vi "MGCC_FntStaMach_Flagtoevent.vi"(9 "M_OFF":bool, 10 "Pre_state":string) -> (2 "Event":bool[](array[boolean]))   [LabVIEW 2016]
uses:
  <vilib>/imath/engines/lvmath/Plug In/_Char/NIMS_CH_character datatype.ctl
  <vilib>/imath/engines/lvmath/Plug In/_Char/NIMS_CH_String to Character Array.vi
  <vilib>/imath/engines/lvmath2/RunTimeEngine/IndexRead/NIMS V(S).vi
  <instcachedir>/0/NIMS V(S)_0488751826AF41519A22953C041130DC.lvgen/NIMS V(S)_0488751826AF41519A22953C041130DC_003.vi
  <vilib>/imath/engines/lvmath2/RunTimeEngine/ErrorHandling/NIMS_Create Error From Enums.vi
  <vilib>/imathl/engines/lvmath/Functions/Error Handling/Create Error.vi
  <vilib>/imath/engines/lvmath2/RunTimeSupport/NIMS_Compare Aggregates.vi
  <instcachedir>/0/NIMS_Compare Aggregates_FA3EBEB3749E48D38A57888B5ABBF163.lvgen/NIMS_Compare Aggregates_FA3EBEB3749E48D38A57888B5ABBF163_000.vi
  <vilib>/imath/engines/lvmath2/RunTimeEngine/VariableToken/NIMS_VariableToken_CondDefined.vi
  <instcachedir>/0/NIMS_VariableToken_CondDefined_06E9DA95BD4D46A6BA55EC651A891960.lvgen/NIMS_VariableToken_CondDefined_06E9DA95BD4D46A6BA55EC651A891960_003.vi
  <vilib>/imath/engines/lvmath2/RunTimeEngine/NodeEndStatement/NIMS_NodeEndStatement_Output.vi
  <instcachedir>/0/NIMS_NodeEndStatement_Output_53EC0D466D134D7ABD903AC30B43404B.lvgen/NIMS_NodeEndStatement_Output_53EC0D466D134D7ABD903AC30B43404B_012.vi
  <vilib>/imath/engines/lvmath2/RunTimeEngine/ErrorHandling/NIMS_Finalize Error.vi
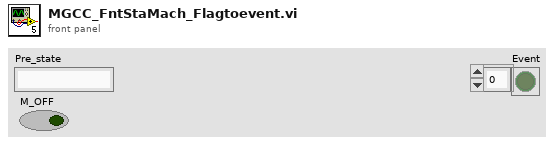
[diagram p1: front panel]
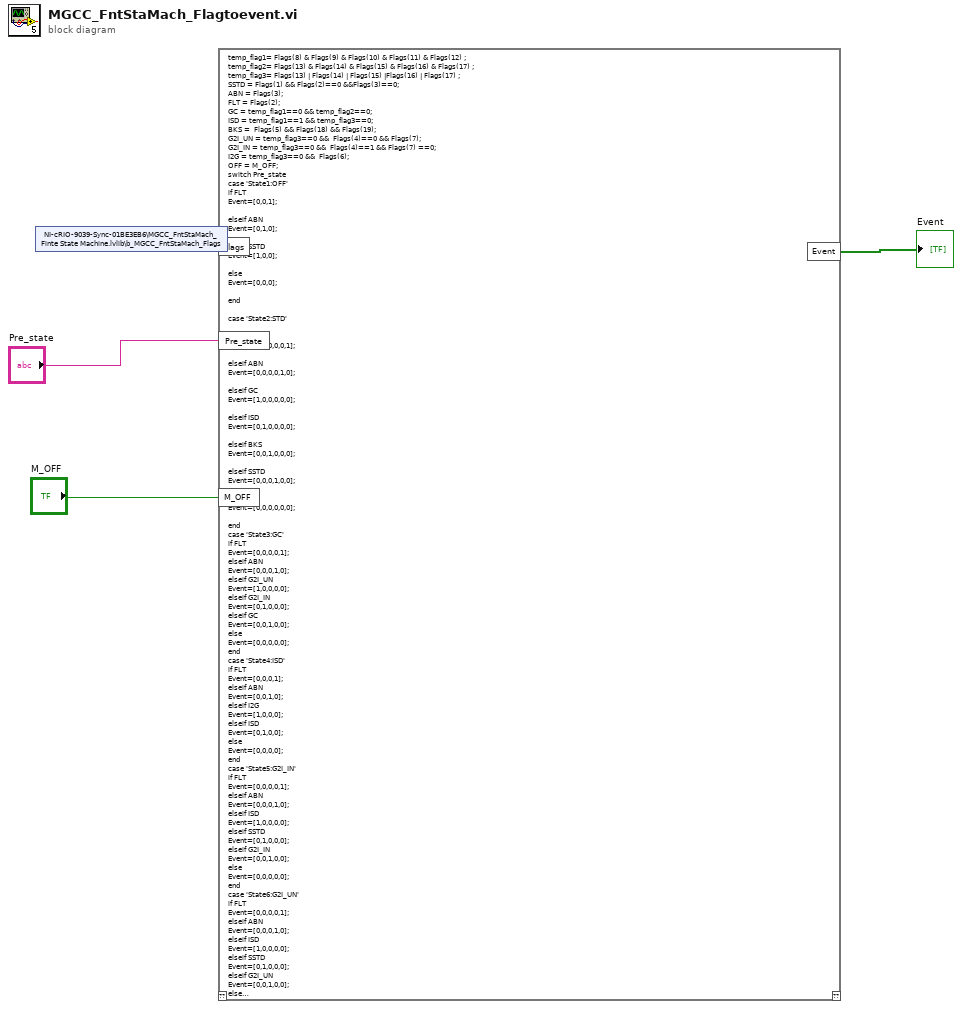
[diagram p0: block diagram]
diagram:
  n1 = shared-variable "NI-cRIO-9039-Sync-01BE3EB6\\MGCC_FntStaMach_Finte State Machine.lvlib\\b_MGCC_FntStaMach_Flags"() -> (w4:bool[])  [unwired: 1 in, 1 out]
  n2 = mathscript code="temp_flag1= Flags(8) & Flags(9) & Flags(10) & Flags(11) & Flags(12) ;\ntemp_flag2= Flags(13) & Flags(14) & Flags(15) & Flags(16) & Flags(17) ;\ntemp_flag3= Flags(13) | Flags(14) | Flags(15) |Flags(16) | Flags(17) ;\nSSTD = Flags(1) && Flags(2)==0 &&Flags(3)==0;\nABN = Flags(3);\nFLT = Flags(2);\nGC = temp_flag1==0 && temp_flag2==0;\nISD = temp_flag1==1 && temp_flag3==0;\nBKS =  Flags(5) && Flags(18) && Flags(19);\nG2I_UN = temp_flag3==0 &&  Flags(4)==0 && Flags(7);\nG2I_IN = temp_flag3==0 &&  Flags(4)==1 && Flags(7) ==0;\nI2G = temp_flag3==0 &&  Flags(6);\nOFF = M_OFF;\nswitch Pre_state\ncase 'State1:OFF'\nif FLT\nEvent=[0,0,1];\n\nelseif ABN\nEvent=[0,1,0];\n\nelseif SSTD\nEvent=[1,0,0];\n\nelse\nEvent=[0,0,0];\n\nend \n\ncase 'State2:STD'\n\nif FLT\nEvent=[0,0,0,0,0,1];\n\nelseif ABN\nEvent=[0,0,0,0,1,0];\n\nelseif GC\nEvent=[1,0,0,0,0,0];\n\nelseif ISD\nEvent=[0,1,0,0,0,0];\n\nelseif BKS\nEvent=[0,0,1,0,0,0];\n\nelseif SSTD\nEvent=[0,0,0,1,0,0];\n\nelse\nEvent=[0,0,0,0,0,0];\n\nend \ncase 'State3:GC'\nif FLT\nEvent=[0,0,0,0,1];\nelseif ABN\nEvent=[0,0,0,1,0];\nelseif G2I_UN\nEvent=[1,0,0,0,0];\nelseif G2I_IN\nEvent=[0,1,0,0,0];\nelseif GC\nEvent=[0,0,1,0,0];\nelse\nEvent=[0,0,0,0,0];\nend\ncase 'State4:ISD'\nif FLT\nEvent=[0,0,0,1];\nelseif ABN\nEvent=[0,0,1,0];\nelseif I2G\nEvent=[1,0,0,0];\nelseif ISD\nEvent=[0,1,0,0];\nelse\nEvent=[0,0,0,0];\nend\ncase 'State5:G2I_IN'\nif FLT\nEvent=[0,0,0,0,1];\nelseif ABN\nEvent=[0,0,0,1,0];\nelseif ISD \nEvent=[1,0,0,0,0];\nelseif SSTD\nEvent=[0,1,0,0,0];\nelseif G2I_IN\nEvent=[0,0,1,0,0];\nelse\nEvent=[0,0,0,0,0];\nend\ncase 'State6:G2I_UN'\nif FLT\nEvent=[0,0,0,0,1];\nelseif ABN\nEvent=[0,0,0,1,0];\nelseif ISD\nEvent=[1,0,0,0,0];\nelseif SSTD\nEvent=[0,1,0,0,0];\nelseif G2I_UN\nEvent=[0,0,1,0,0];\nelse\nEvent=[0,0,0,0,0];\nend\ncase 'State7:I2G'\nif FLT\nEvent=[0,0,0,0,1];\nelseif ABN\nEvent=[0,0,0,1,0];\nelseif GC\nEvent=[1,0,0,0,0];\nelseif SSTD\nEvent=[0,1,0,0,0];\nelseif I2G\nEvent=[0,0,1,0,0];\nelse\nEvent=[0,0,0,0,0];\nend\ncase 'State8:BKS'\nif FLT\nEvent=[0,0,0,0,1];\nelseif ABN\nEvent=[0,0,0,1,0];\nelseif ISD\nEvent=[1,0,0,0,0];\nelseif SSTD\nEvent=[0,1,0,0,0];\nelseif BKS\nEvent=[0,0,1,0,0];\nelse\nEvent=[0,0,0,0,0];\nend\ncase 'State9:ABN'\nif FLT\nEvent=[0,0,0,0,0,0,0,0,1];\nelseif ABN\nEvent=[0,0,0,0,0,0,0,1,0];\nelseif SSTD\nEvent=[1,0,0,0,0,0,0,0,0];\nelseif GC\nEvent=[0,1,0,0,0,0,0,0,0];\nelseif ISD\nEvent=[0,0,1,0,0,0,0,0,0];\nelseif G2I_UN\nEvent=[0,0,0,1,0,0,0,0,0];\nelseif G2I_IN\nEvent=[0,0,0,0,1,0,0,0,0];\nelseif I2G\nEvent=[0,0,0,0,0,1,0,0,0];\nelseif BKS\nEvent=[0,0,0,0,0,0,1,0,0];\nelse\nEvent=[0,0,0,0,0,0,0,0,0];\nend\ncase 'State10:FLT'\nif FLT\nEvent=[1,0,0,0];\nelseif ABN\nEvent=[0,1,0,0];\nelseif SSTD\nEvent=[0,0,1,0];\nelseif OFF\nEvent=[0,0,0,1];\nelse\nEvent=[0,0,0,0];\nend\notherwise\nend"("Flags"=w4, "Pre_state"="Pre_state", "M_OFF"="M_OFF") -> ("Event"=→"Event":bool[])  [unwired: 1 in, 1 out]
